vi "uServices Replies Check.vi"(8 "error in (no error)":errorcluster, 11 "Tamer in":refnum<class "Tamer.lvclass">) -> (0 "error out":errorcluster, 3 "Tamer out":refnum<class "Tamer.lvclass">)   [LabVIEW 2020, in "TALOS.lvlib" / "Tamer.lvlib" / "Tamer.lvclass"]
uses:
  Tamer.lvclass
  C:/LabVIEW Code/TALOS/talos/Father of all uServices/Father of all uServices/Father of all uServices.lvclass
  Tamer.lvclass/Tamer.ctl
  Ancestor/Ancestor/Ancestor.lvclass/Ancestor.ctl
  Tamer Consumer Case Selector.ctl
  Father of all uServices/Father of all uServices Messages/Consumer Msg/Consumer Msg.lvclass/Consumer Msg.ctl
  1a23463c-f434-4530-8538-5d2d60edc9f3.vi
  b26088c6-870e-48d3-b395-768c6d5583f0.vi
  c4765a06-6b21-48d1-820a-4616241c9526.vi
  cc401d95-25fb-404c-8af8-60e8e1838a9f.vi
  b26088c6-870e-48d3-b395-768c6d5583f0.vi/c0db33a9-eb6c-44d9-b982-8563e05d2734.vi
  b26088c6-870e-48d3-b395-768c6d5583f0.vi/ae3535a8-0066-4e8d-a5de-b07ac05a7c65.vi
  b26088c6-870e-48d3-b395-768c6d5583f0.vi/dda8e586-731b-4197-ad83-6a4d05585a0a.vi
  c4765a06-6b21-48d1-820a-4616241c9526.vi/c0db33a9-eb6c-44d9-b982-8563e05d2734.vi
  c4765a06-6b21-48d1-820a-4616241c9526.vi/ae3535a8-0066-4e8d-a5de-b07ac05a7c65.vi
  c4765a06-6b21-48d1-820a-4616241c9526.vi/dda8e586-731b-4197-ad83-6a4d05585a0a.vi
  FGV/Error Memory/Get Error Description.vi
  Support VIs/Get PC name.vi
  Ancestor/Ancestor/Read ID.vi
  Support VIs/Get Class Name.vi
  <vilib>/Utility/error.llb/Clear Errors.vi
  Father of all uServices/Father of all uServices Messages/Consumer Msg/Send Consumer.vi
  FGV/Error Memory/Error Memory Core.vi
  <vilib>/AdvancedString/Delimited String to 1D String Array.vi
  Support VIs/Circus Root Path.vi
  FGV/Error Memory/Error Crt Lvl checker.vi
  FGV/Error Memory/Error Memory Core.vi/40c8088d-b597-4017-91af-faa98e00292e.vi
  FGV/Error Memory/Error Memory Core.vi/d4a3ab98-063c-4e44-b43d-fbdcfe6c2be2.vi
  Father of all uServices/Father of all uServices/Father of all uServices.lvclass
  C:/LabVIEW Code/TALOS/builds/Actor Framework PPL/Actor Framework.lvlibp/1abvi3w/vi.lib/ActorFramework/Actor/Actor.lvclass
  Support VIs/Global Memory.vi
  <vilib>/Utility/LVClass/Get LV Class Name.vi
  Support VIs/Is in Packed Library.vi
  Support VIs/TALOS Root path.vi
  Support VIs/Read CSV worksheet.vi
  Support VIs/Global Constants.vi
  <vilib>/Utility/error.llb/General Error Handler.vi
  Support VIs/Error Log.vi
  builds/Actor Framework PPL/Actor Framework.lvlibp/1abvi3w/vi.lib/ActorFramework/Actor/Read Self Enqueuer.vi
  <userlib>/_OpenG.lib/lvdata/lvdata.llb/Get Strings from Enum__ogtk.vi
  builds/Actor Framework PPL/Actor Framework.lvlibp/1abvi3w/vi.lib/ActorFramework/Message Enqueuer/Enqueue.vi
  <vilib>/Comparison/Less/Less Functor/Less Functor.lvclass
  Ancestor/Ancestor/Ancestor.lvclass
  <vilib>/Comparison/Equal/Equal Functor/Equal Functor.lvclass
  Father of all uServices/Father of all uServices Messages/Consumer Msg/Consumer Msg.lvclass
  TALOS.lvlib
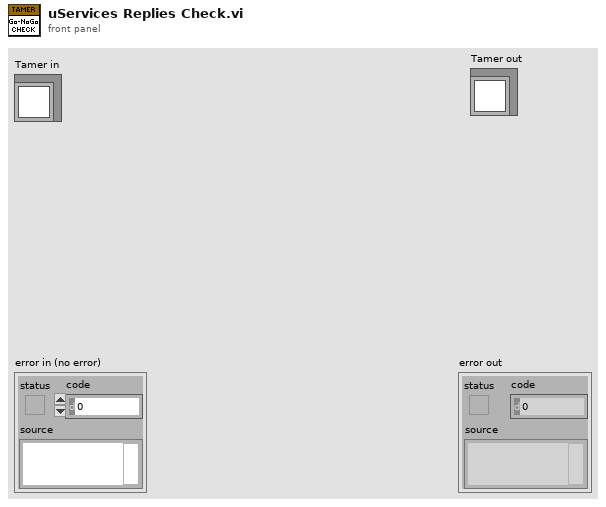
[diagram p1: front panel]
types:
  T1 = typedef "TALOS.lvlib/Tamer.lvlib/Tamer.lvclass/Tamer Consumer Case Selector.ctl" = enum16{"New schedule", "Initiate RUN", "Parse Schedules", "Script Checker", "Banana after Quality Check", "Update Crit Lvl", "Propagate Banana", "Reply from Guardian", "Reply from uService", "Timeout of RUN", "uService Replies Check", "Update from Monkey", "Monkey Died", "Reschedule", "Rerun", "Stop DAQ", "Stop Schedule", "Skip Run", "Kill Process", "Update GV"}
  T2 = typedef "TALOS.lvlib/Tamer.lvlib/Tamer.lvclass/Reply.ctl" = cluster{"ID":string, "Status":bool, "GUID":string}
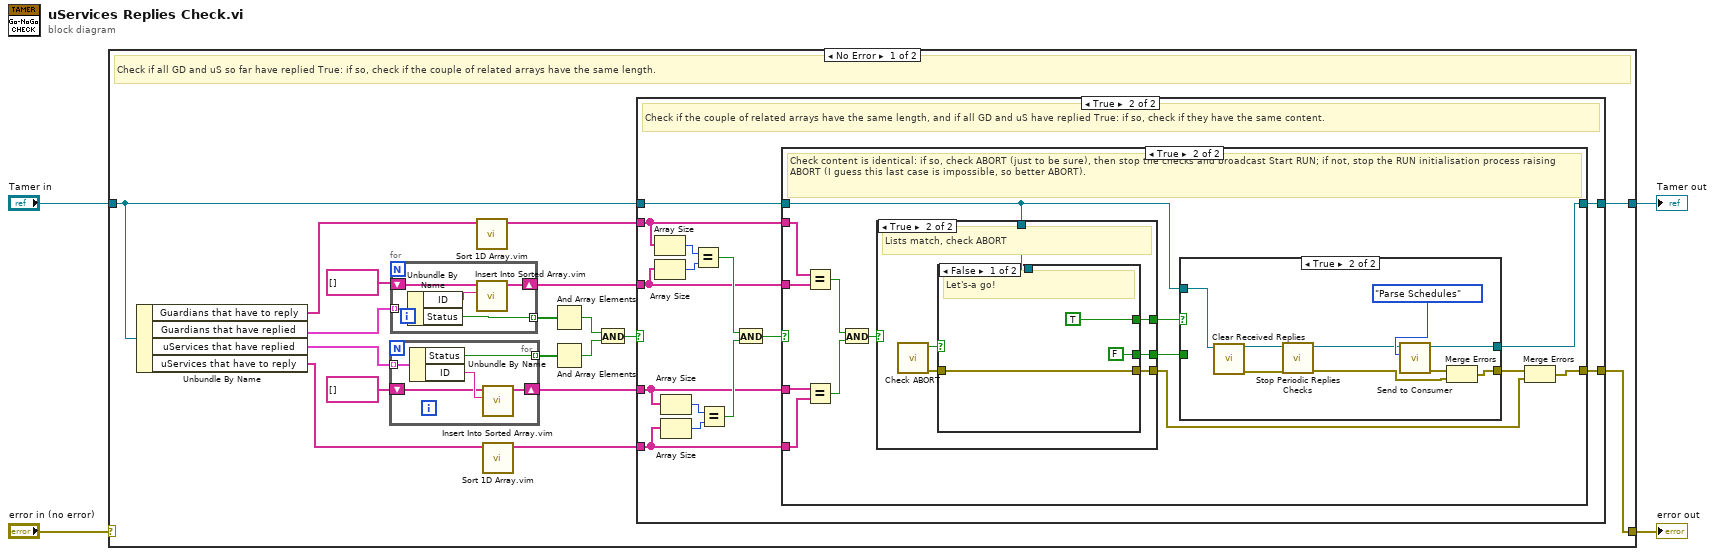
[diagram p0: block diagram]
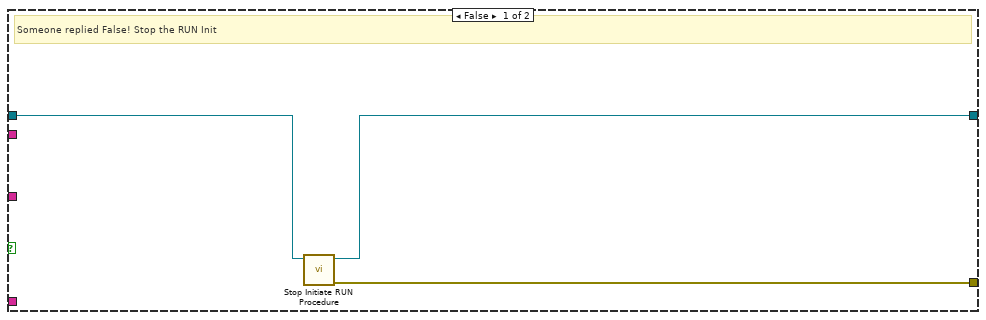
[diagram p2: hidden frame]
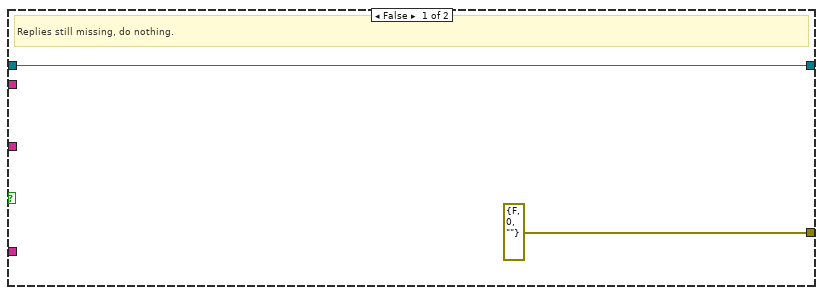
[diagram p3: hidden frame]
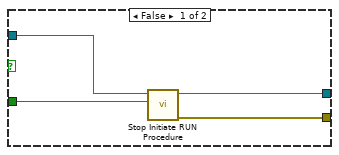
[diagram p4: hidden frame]
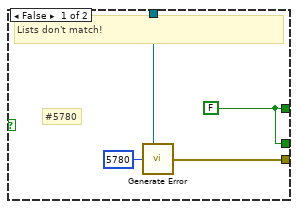
[diagram p5: hidden frame]
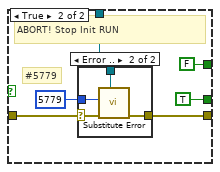
[diagram p6: hidden frame]
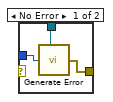
[diagram p7: hidden frame]
diagram:
  n1 = case shown="No Error" "error in (no error)" {
    selector: "error in (no error)" -> [_ w106]
    tunnel: [w20 w106] -> w3
    tunnel: [w21 w105] -> w1
    tunnel: "Tamer in" -> [w22 w105]
    frame No Error {
      # "Check if all GD and uS so far have replied True: if so, check if the couple of related arrays have the same length."
      n2 = Unbundle By Name(w22) -> ("Guardians that have to reply"=w9:string[], "Guardians that have replied"=w19:T2[], "uServices that have replied"=w13:T2[], "uServices that have to reply"=w5:string[])
      n3 = for {
        tunnel: w13 -> [w27] mode=indexing
        tunnel: [w26] -> w15 mode=indexing
        shift-right: [w23] -> w12
        shift-left: string[] [] ("Guardians that have to reply") -> [w24]
        n4 = Unbundle By Name(w27) -> ("Status"=w26:bool, "ID"=w25:string)
        n5 = call "Insert Into Sorted Array.vim"("element"=w25, "sorted array in"=w24) -> ("sorted array out"=w23:string[])  [unwired: 9 in]
      }
      n6 = for {
        tunnel: w19 -> [w32] mode=indexing
        tunnel: [w31] -> w14 mode=indexing
        shift-right: [w28] -> w10
        shift-left: string[] [] ("Guardians that have to reply") -> [w29]
        n7 = Unbundle By Name(w32) -> ("ID"=w30:string, "Status"=w31:bool)
        n8 = call "Insert Into Sorted Array.vim"("element"=w30, "sorted array in"=w29) -> ("sorted array out"=w28:string[])  [unwired: 9 in]
      }
      n9 = call "Sort 1D Array.vim"("unsorted array"=w9) -> ("sorted array"=w8:string[])  [unwired: 10 in]
      n10 = call "Sort 1D Array.vim"("unsorted array"=w5) -> ("sorted array"=w6:string[])  [unwired: 10 in]
      n11 = And Array Elements(Boolean array=w14) -> (logical AND=w17:bool)
      n12 = And Array Elements(Boolean array=w15) -> (logical AND=w16:bool)
      n13 = And(x=w17, y=w16) -> (x .and. y?=w18:bool)
      n14 = case shown="True" w18 {
        tunnel: w8 -> [_ w36]
        tunnel: w22 -> [w35 w45]
        tunnel: [w34 w44] -> w21
        tunnel: [w33 w43] -> w20
        tunnel: w6 -> [_ w38]
        tunnel: w10 -> [_ w37]
        tunnel: w12 -> [_ w39]
        frame False {
          # "Someone replied False! Stop the RUN Init"
          n15 = call "Stop Initiate RUN Procedure.vi"("Tamer in"=w35) -> ("error out"=w33:errorcluster, "Tamer out"=w34:refnum<class "Tamer.lvclass">)  [unwired: 9 in]
        }
        frame True {
          # "Check if the couple of related arrays have the same length, and if all GD and uS have replied True: if so, check if they have the same content."
          n16 = Array Size(array=w36) -> (size(s)=w41:i32)
          n17 = Array Size(array=w37) -> (size(s)=w42:i32)
          n18 = Array Size(array=w39) -> (size(s)=w49:i32)
          n19 = Array Size(array=w38) -> (size(s)=w48:i32)
          n20 = Equal?(x=w41, y=w42) -> (x = y?=w40:bool)
          n21 = Equal?(x=w49, y=w48) -> (x = y?=w47:bool)
          n22 = And(x=w40, y=w47) -> (x .and. y?=w46:bool)
          n23 = case shown="True" w46 {
            tunnel: w45 -> [w51 w63]
            tunnel: [w51 w64] -> w44
            tunnel: [errorcluster {"status"=FALSE, "code"=0, "source"=""} ("error out") w58] -> w43
            tunnel: w39 -> [_ w54]
            tunnel: w38 -> [_ w55]
            tunnel: w37 -> [_ w53]
            tunnel: w36 -> [_ w52]
            frame False {
              # "Replies still missing, do nothing."
            }
            frame True {
              # "Check content is identical: if so, check ABORT (just to be sure), then stop the checks and broadcast Start RUN; if not, stop the RUN initialisation process raising ABORT (I guess this last case is impossible, so better ABORT)."
              n24 = Equal?(x=w52, y=w53) -> (x = y?=w62:bool)
              n25 = Equal?(x=w54, y=w55) -> (x = y?=w60:bool)
              n26 = And(x=w62, y=w60) -> (x .and. y?=w61:bool)
              n27 = case shown="True" w61 {
                tunnel: [w81 w86] -> w57
                tunnel: w63 -> [w80 w85]
                tunnel: [w79 w84] -> w59
                tunnel: [w79 w83] -> w56
                frame False {
                  w79 = FALSE
                  # "#5780"
                  # "Lists don't match!"
                  n28 = call "Generate Error.vi"("Class"=w80, "Error Code"=5780) -> ("error out"=w81:errorcluster)  [unwired: 5 in]
                }
                frame True {
                  # "Lists match, check ABORT"
                  n29 = call "Check ABORT.vi"() -> ("error out"=w88:errorcluster, "ABORT?"=w87:bool)  [unwired: 10 in]
                  n30 = case shown="False" w87 {
                    tunnel: w88 -> [w91 w97]
                    tunnel: [w91 w95] -> w86
                    tunnel: w85 -> [_ w94]
                    tunnel: [TRUE FALSE] -> w84
                    tunnel: [FALSE TRUE] -> w83
                    frame False {
                      # "Let's-a go!"
                    }
                    frame True {
                      # "#5779"
                      # "ABORT! Stop Init RUN"
                      n31 = case shown="Error .." w97 {
                        selector: w97 -> [_ w104]
                        tunnel: 5779 ("Error Code") -> [w100 w103]
                        tunnel: [w99 w102] -> w95
                        tunnel: w94 -> [w98 w101]
                        frame No Error {
                          n32 = call "Generate Error.vi"("Class"=w98, "Error Code"=w100) -> ("error out"=w99:errorcluster)  [unwired: 5 in]
                        }
                        frame Error {
                          n33 = call "Substitute Error.vi"("LabVIEW Object"=w101, "error in (no error)"=w104, "Error Code"=w103) -> ("error out"=w102:errorcluster)  [unwired: 8 in]
                        }
                      }
                    }
                  }
                }
              }
              n34 = case shown="True" w59 {
                tunnel: w63 -> [w68 w75]
                tunnel: [w69 w76] -> w65
                tunnel: [w67 w78] -> w64
                tunnel: w56 -> [w66 _]
                frame False {
                  n35 = call "Stop Initiate RUN Procedure.vi"("Stop for good"=w66, "Tamer in"=w68) -> ("error out"=w69:errorcluster, "Tamer out"=w67:refnum<class "Tamer.lvclass">)  [unwired: 8 in]
                }
                frame True {
                  n36 = call-dynamic "Clear Received Replies.vi"("Tamer in"=w75) -> ("error out"=w72:errorcluster, "Tamer out"=w73:refnum<class "Tamer.lvclass">)  [unwired: 9 in]
                  n37 = call-dynamic "Stop Periodic Replies Checks.vi"("error in (no error)"=w72, "Tamer in"=w73) -> ("error out"=w71:errorcluster, "Tamer out"=w70:refnum<class "Tamer.lvclass">)  [unwired: 8 in]
                  n38 = call "Send to Consumer.vi"("Case ID"=Tamer_Consumer_Case_Selector."Parse Schedules" ("Monkey Consumer Case Selector"), "uService Template in"=w70) -> ("error out"=w77:errorcluster, "uService Template out"=w78:refnum<class "Tamer.lvclass">)  [unwired: 8 in]
                  n39 = Merge Errors(w77, w71) -> (w76:errorcluster)
                }
              }
              n40 = Merge Errors(w65, w57) -> (w58:errorcluster)
            }
          }
        }
      }
    }
    frame Error {
    }
  }
  "error out" <- w3
  "Tamer out" <- w1
